vi "tstp_can_send_functional.vi"(8 "error in (no error)":errorcluster, 9 "Data":u8[](array[numeric]), 10 "ADiagModuleIndex":i32, 11 "路径输入":path) -> (0 "error out":errorcluster, 2 "return":i32, 3 "路径输出":path)   [LabVIEW 2014]
doc: "根据功能地址Request ID发送数据。"
panel:
  out "Succes？":bool
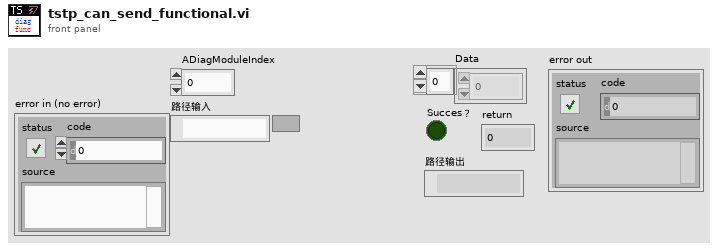
[diagram p1: front panel]
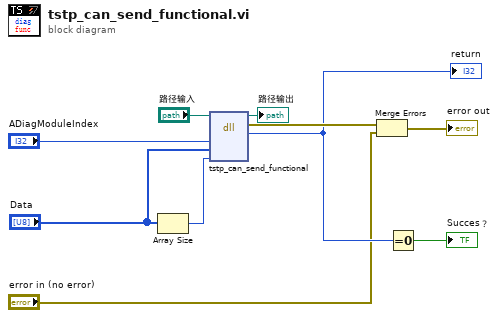
[diagram p0: block diagram]
diagram:
  n1 = Array Size(array="Data") -> (size(s)=w4:i32)
  n2 = dll-call lib="D:/Program Files (x86)/TOSUN/TSMaster/bin/TSMaster.dll" fn="tstp_can_send_functional"(path in="路径输入", "ADiagModuleIndex"="ADiagModuleIndex", "AReqDataArray"="Data", "AReaDataSize"=w4) -> (path out=→"路径输出":path, error out=w10:errorcluster, "ACode"=w7:i32)  [unwired: 5 in]
  "return" <- w7
  n3 = Merge Errors(w10, "error in (no error)") -> (→"error out":errorcluster)
  n4 = Equal To 0?(x=w7) -> (x = 0?=→"Succes？":bool)
